vi "发送串口数据.vi"(8 "error in (no error)":errorcluster caption="错误输入（无错误）", 10 "原始数据":string, 11 "硬件 输入":refnum<class "硬件.lvclass">) -> (0 "error out":errorcluster caption="错误输出", 2 "已发送":string, 3 "硬件 输出":refnum<class "硬件.lvclass">)   [LabVIEW 2015, in "硬件.lvlib" / "硬件.lvclass"]
uses:
  <vilib>/Instr/_visa.llb/VISA Configure Serial Port (Instr).vi
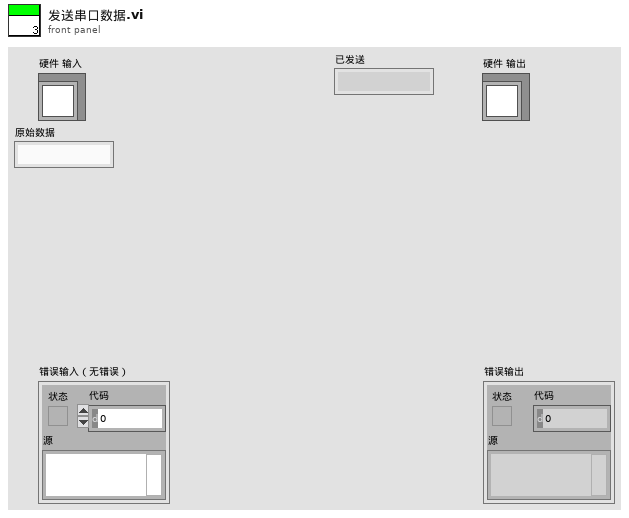
[diagram p1: front panel]
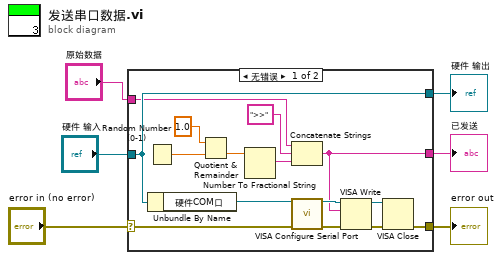
[diagram p0: block diagram]
diagram:
  n1 = case shown="无错误" "error in (no error)" {
    selector: "error in (no error)" -> [w19 w24]
    tunnel: [w13 w24] -> w5
    tunnel: [w21 w23] -> w3
    tunnel: "硬件 输入" -> [w21 w23]
    tunnel: "原始数据" -> [w16 w22]
    tunnel: [w11 w22] -> w1
    frame No Error {
      n2 = Random Number (0-1)() -> (number: 0 to 1=w9:dbl)
      n3 = Unbundle By Name(w21) -> ("硬件COM口"=w20:refnum<visa-resource-name>)
      n4 = Quotient & Remainder(x=1.0, y=w9) -> (floor(x/y)=w8:dbl)  [unwired: 1 out]
      n5 = Number To Fractional String(number=w8) -> (F-format string=w7:string)  [unwired: 3 in]
      n6 = Concatenate Strings(w16, ">>" ("字符串"), w7) -> (w11:string)
      n7 = call-poly "VISA Configure Serial Port"("VISA resource name"=w20, "error in (no error)"=w19) -> ("VISA resource name out"=w18:refnum<visa-resource-name>, "error out"=w17:errorcluster)  [unwired: 12 in]
      n8 = VISA Write(VISA resource name=w18, write buffer=w11, error in (no error)=w17) -> (VISA resource name out=w15:refnum<visa-resource-name>, error out=w14:errorcluster)  [unwired: 1 out]
      n9 = VISA Close(VISA resource name=w15, error in (no error)=w14) -> (error out=w13:errorcluster)
    }
    frame Error {
    }
  }
  "error out" <- w5
  "硬件 输出" <- w3
  "已发送" <- w1
